vi "Increment Timestamp.vi"(2 "Days":i32, 3 "Time Stamp":timestamp) -> (1 "Time Stamp out":timestamp)   [LabVIEW 2020, in "ARecurrence.lvclass"]
uses:
  ARecurrence.lvclass
  ARecurrence.lvclass/ARecurrence.ctl
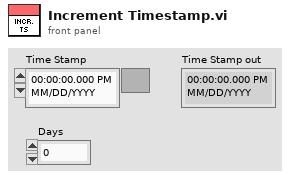
[diagram p1: front panel]
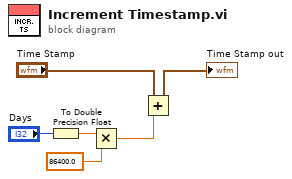
[diagram p0: block diagram]
diagram:
  n1 = To Double Precision Float(number="Days") -> (double precision float=w5:dbl)
  n2 = Multiply(x=w5, y=86400.0) -> (x*y=w2:dbl)
  n3 = Add(x="Time Stamp", y=w2) -> (x+y=→"Time Stamp out":timestamp)
